vi "S2C_FORNAX_Proc_InitGlobals.vi"(8 "Error In":errorcluster) -> (0 "Error Out":errorcluster)   [LabVIEW 2015]
uses:
  S2C_FORNAX_Proc_Globals.vi
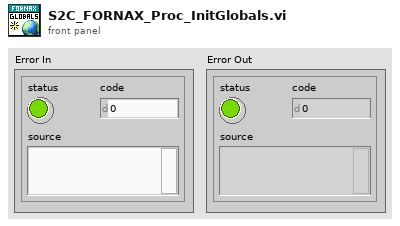
[diagram p1: front panel]
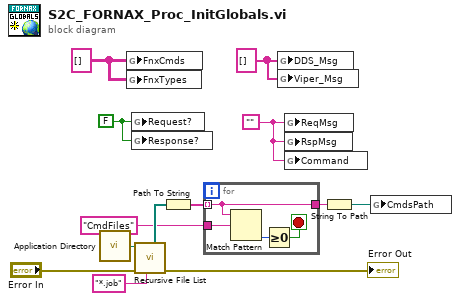
[diagram p0: block diagram]
diagram:
  w10 = FALSE ("Request?")
  w11 = ""
  w12 = string[] [] ("DDS_Msg")
  w13 = string[][][] [] ("FnxCmds")
  n1 = call <vilib>:"Application Directory.vi"() -> ("Application Directory"=w8:path)
  n2 = global write "S2C_FORNAX_Proc_Globals.vi" "FnxCmds"(w13) -> ()
  n3 = global write "S2C_FORNAX_Proc_Globals.vi" "FnxTypes"(w13) -> ()
  n4 = global write "S2C_FORNAX_Proc_Globals.vi" "Request?"(w10) -> ()
  n5 = global write "S2C_FORNAX_Proc_Globals.vi" "Response?"(w10) -> ()
  n6 = call <vilib>:"Recursive File List.vi"("pattern"="*.job", "error in (no error)"="Error In", "Folder Path"=w8) -> ("error out"=→"Error Out":errorcluster, "All Folders"=w6:path[])  [unwired: 4 in, 3 out]
  n7 = Path To String(path=w6) -> (string=w5:string[])
  n8 = for {
    tunnel: w5 -> [w14] mode=indexing
    tunnel: "CmdFiles" ("regular expression") -> [w17]
    tunnel: [w14] -> w3
    stop <- w15 stop-if-true
    n9 = Match Pattern(string=w14, regular expression=w17) -> (offset past match=w16:i32)  [unwired: 1 in, 3 out]
    n10 = Greater Or Equal To 0?(x=w16) -> (x >= 0?=w15:bool)
  }
  n11 = global write "S2C_FORNAX_Proc_Globals.vi" "DDS_Msg"(w12) -> ()
  n12 = global write "S2C_FORNAX_Proc_Globals.vi" "Viper_Msg"(w12) -> ()
  n13 = global write "S2C_FORNAX_Proc_Globals.vi" "ReqMsg"(w11) -> ()
  n14 = global write "S2C_FORNAX_Proc_Globals.vi" "RspMsg"(w11) -> ()
  n15 = global write "S2C_FORNAX_Proc_Globals.vi" "Command"(w11) -> ()
  n16 = String To Path(string=w3) -> (path=w2:path)
  n17 = global write "S2C_FORNAX_Proc_Globals.vi" "CmdsPath"(w2) -> ()
